vi "Test Tag Read FLAC.vi"(8 "error in (no error)":errorcluster) -> (0 "error out":errorcluster, 3 "Pass?":bool)   [LabVIEW 2020]
uses:
  G-Audio/Audio Files/Polymorphic VIs/Get Audio File Tags (Path).vi
  G-Audio/G-Audio.lvlib
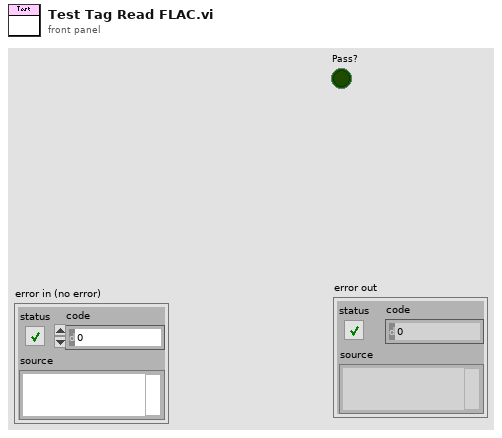
[diagram p1: front panel]
types:
  T1 = typedef "G-Audio.lvlib/Audio File Tag.ctl" = cluster{"Field":string, "Value":string}
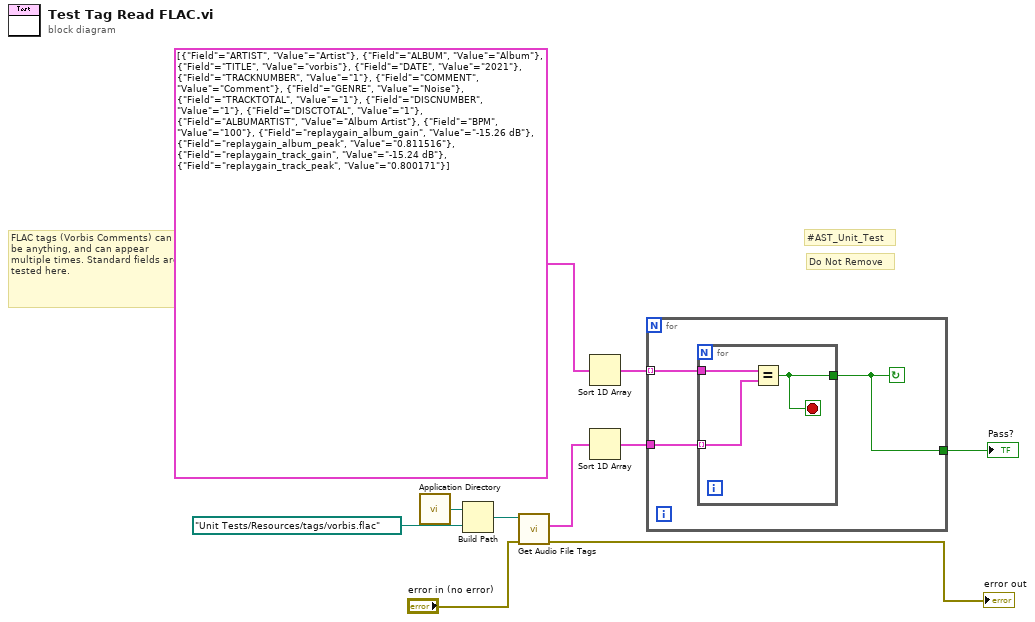
[diagram p0: block diagram]
diagram:
  # "FLAC tags (Vorbis Comments) can be anything, and can appear multiple times. Standard fields are tested here."
  # "Do Not Remove"
  # "#AST_Unit_Test"
  n1 = call <vilib>:"Application Directory.vi"() -> ("Application Directory"=w10:path)
  n2 = Build Path(base path=w10, name or relative path=path "Unit Tests/Resources/tags/vorbis.flac" ("Path")) -> (appended path=w8:path)
  n3 = call-poly "Get Audio File Tags.vi"("error in (no error)"="error in (no error)", "Path In"=w8) -> ("error out"=→"error out":errorcluster, "Tags"=w5:T1[])  [unwired: 6 in, 2 out]
  n4 = Sort 1D Array(array=cluster{"Field":string, "Value":string}[] [{"Field"="ARTIST", "Value"="Artist"}, {"Field"="ALBUM", "Value"="Album"}, {"Field"="TITLE", "Value"="vorbis"}, {"Field"="DATE", "Value"="2021"}, {"Field"="TRACKNUMBER", "Value"="1"}, {"Field"="COMMENT", "Value"="Comment"}, {"Field"="GENRE", "Value"="Noise"}, {"Field"="TRACKTOTAL", "Value"="1"}, {"Field"="DISCNUMBER", "Value"="1"}, {"Field"="DISCTOTAL", "Value"="1"}, {"Field"="ALBUMARTIST", "Value"="Album Artist"}, {"Field"="BPM", "Value"="100"}, {"Field"="replaygain_album_gain", "Value"="-15.26 dB"}, {"Field"="replaygain_album_peak", "Value"="0.811516"}, {"Field"="replaygain_track_gain", "Value"="-15.24 dB"}, {"Field"="replaygain_track_peak", "Value"="0.800171"}]) -> (sorted array=w3:cluster{"Field":string, "Value":string}[])
  n5 = Sort 1D Array(array=w5) -> (sorted array=w4:T1[])
  n6 = for {
    tunnel: w4 -> [w13]
    tunnel: w3 -> [w11] mode=indexing
    tunnel: [w12] -> w1
    stop <- w12 continue-if-true
    n7 = for {
      tunnel: w13 -> [w14] mode=indexing
      tunnel: [w15] -> w12
      tunnel: w11 -> [w16]
      stop <- w15 stop-if-true
      n8 = Equal?(x=w16, y=w14) -> (x = y?=w15:bool)
    }
  }
  "Pass?" <- w1
